vi "libdaq_gpio_get_iocount.vi"(0 "error in (no error)":errorcluster, 1 "device_name":string, 2 "module_name":string) -> (14 "error out":errorcluster, 15 "device_name":string, 16 "module_name":string, 18 "iocount":u8)   [LabVIEW 2010, in "libdaqVI.lvlib"]
doc: "获取连接到计算机系统上的DAQ设备的数量"
uses:
  libdaqVI.lvlib
  dll/daqlib.dll
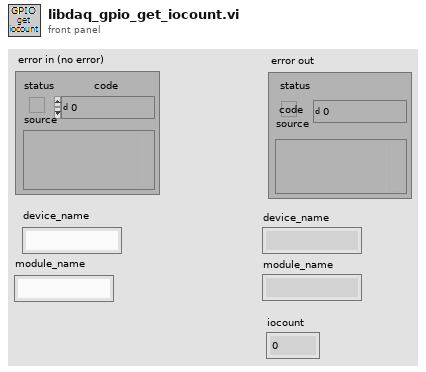
[diagram p1: front panel]
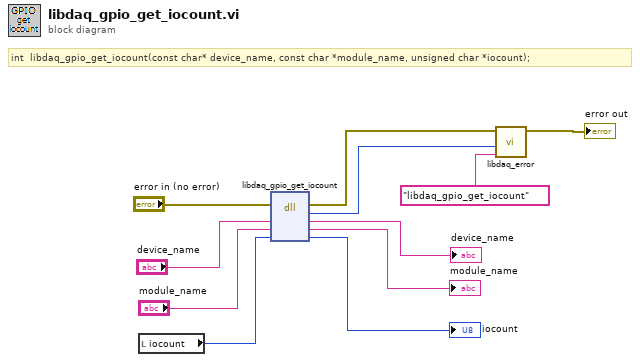
[diagram p0: block diagram]
diagram:
  # "int  libdaq_gpio_get_iocount(const char* device_name, const char *module_name, unsigned char *iocount);"
  n1 = local read "iocount"() -> (w8:u8)
  n2 = dll-call lib="E:/Product/Example/DAQ-USB3212/Labview/labview_2010/libdaqVI/dll/daqlib.dll" fn="libdaq_gpio_get_iocount"(error in="error in (no error)", "device_name"="device_name", "module_name"="module_name", "iocount"=w8) -> (error out=w6:errorcluster, "return type"=w4:i32, "device_name"=→"device_name":string, "module_name"=→"module_name":string, "iocount"=→"iocount":u8)  [unwired: 2 in, 1 out]
  n3 = call "libdaq_error.vi"("error source"="libdaq_gpio_get_iocount", "error code"=w4, "错误输入（无错误）"=w6) -> ("错误输出"=→"error out":errorcluster)  [unwired: 8 in]
